vi "Test1_3.vi"(7 "Report Enable":bool, 8 "error in":errorcluster, 9 "Cycles Burst":i32=10000, 10 "DT_50_L0":i32[][](array[numeric]), 11 "Instrument VISA in":T1={"AWG VISA"="81160A", "Oscilloscope  VISA "="DSO80204B", "Integration Board IP"="172.16.7.43", "connection ID"=refnum, "report out"=refnum}) -> (0 "error out":errorcluster, 2 "L1_Calibration":dbl[][](array[numeric]), 3 "Instrument VISA out":T1={"AWG VISA"="81160A", "Oscilloscope  VISA "="DSO80204B", "Integration Board IP"="172.16.7.43", "connection ID"=refnum, "report out"=refnum})   [LabVIEW 2009]
doc: "This VI does a L1 calibration using different modes depending on the number of pixels active."
uses:
  <instrlib>/Agilent 81150/Agilent 81150.lvlib
  <vilib>/Analysis/NI_AALPro.lvlib
  <vilib>/Utility/NIReport.llb/NI_report.lvclass
  <vilib>/Utility/NIReport.llb/Append Text Table to Report (wrap).vi
  <vilib>/Utility/NIReport.llb/Append Report Text (str wrap).vi
panel:
  out "XY Graph":cluster{"Y":dbl[], "Y":dbl[]}[](graph)
  # "Mode"
  # "Row"
  # "Column"
  # "Number of pixels active"
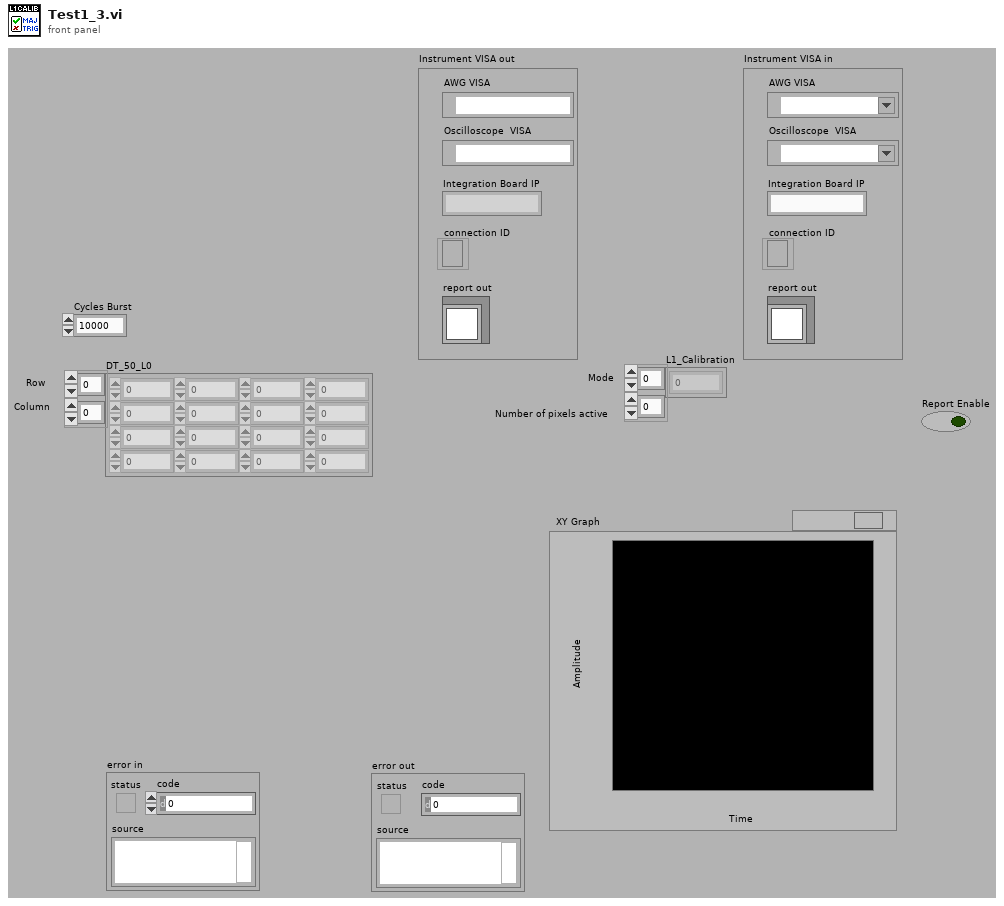
[diagram p1: front panel]
types:
  T1 = cluster{"AWG VISA":refnum<visa-resource-name>, "Oscilloscope  VISA ":refnum<visa-resource-name>, "Integration Board IP":string, "connection ID":refnum<k5>, "report out":refnum<class "NI_report.lvclass">}
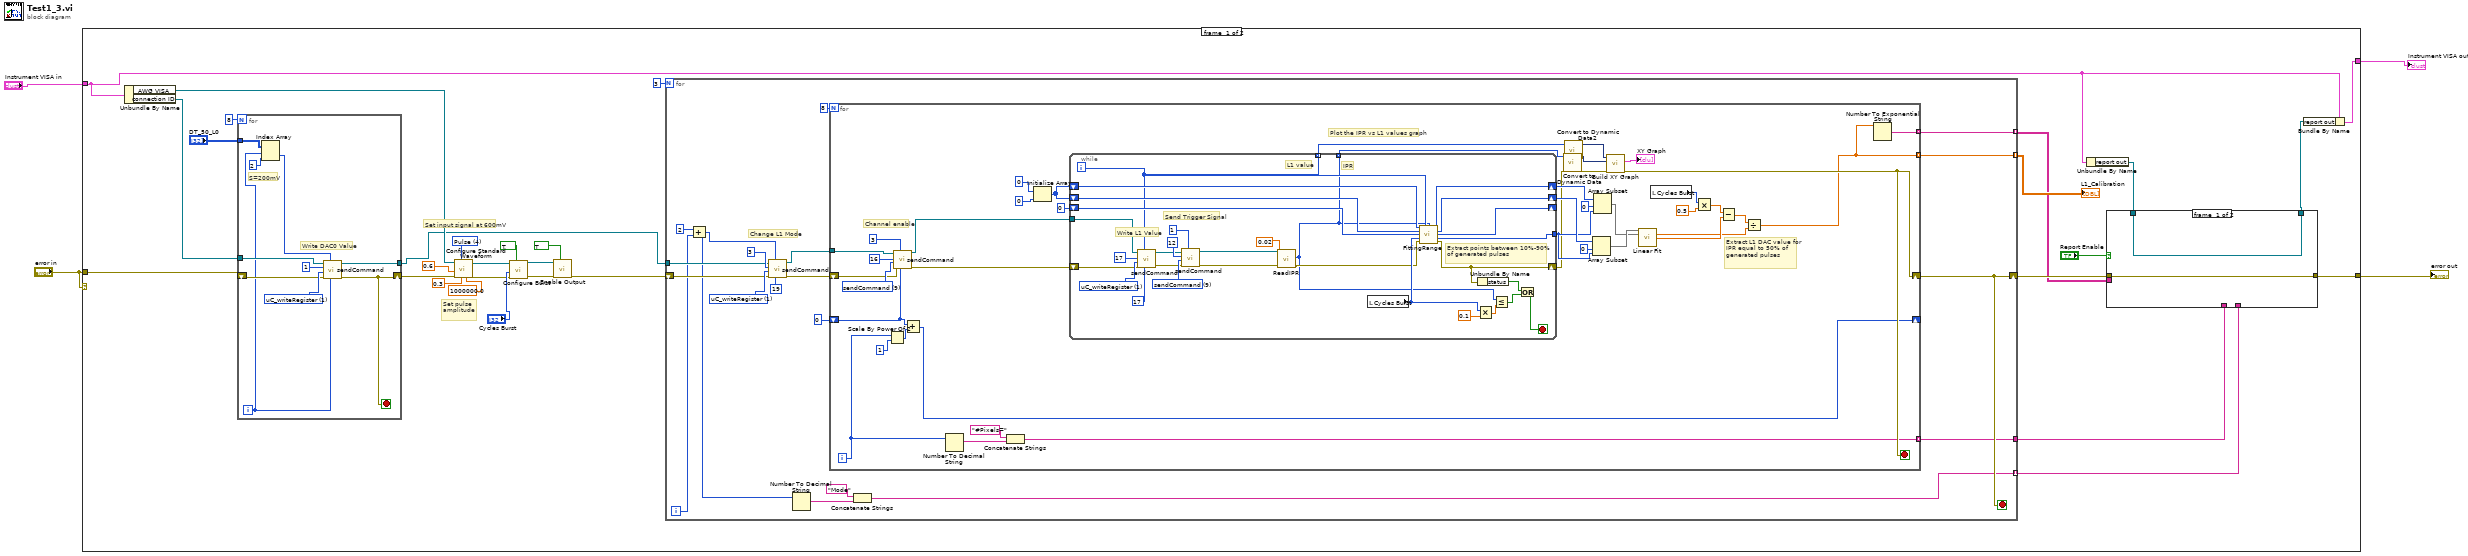
[diagram p0: block diagram]
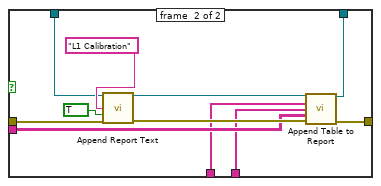
[diagram p2: hidden frame]
diagram:
  n1 = case shown="No Error" "error in" {
    tunnel: "error in" -> [w32 w150]
    tunnel: "Instrument VISA in" -> [w7 w149]
    tunnel: [w14 w150] -> w3
    tunnel: [w6 w149] -> w1
    frame #0 {
      w30 = u16 4 items=["Sine", "Square", "Ramp Up", "Ramp Down", "Pulse", "Noise", "DC"] ("Waveform (0: Sine)")
      # "Set input signal at 600mV"
      # "Set pulse amplitude"
      n2 = Unbundle By Name(w7) -> ("AWG VISA"=w27:refnum<visa-resource-name>, "connection ID"=w33:refnum<k5>)
      n3 = for {
        N: 8 -> [_]
        shift-right: [w139] -> w28
        shift-left: w32 -> [w145]
        tunnel: w33 -> [w143]
        tunnel: "DT_50_L0" -> [w146]
        tunnel: [w140] -> w17
        i -> [w141]
        stop <- w139 stop-if-true
        w148 = u16 1 items=["sendCommand"=9, "FPGA_writeRegister"=3, "FPGA_readRegister"=2, "uC_writeRegister"=1, "uC_readRegister"=0] ("Action")
        # "S=200mV"
        # "Write DAC0 Value"
        n4 = Index Array(array=w146, index (row)=w141, index (col)=2 ("disabled index (col)")) -> (element=w144:i32)
        n5 = call "sendCommand.vi"("Address"=w141, "Data"=w144, "error in"=w145, "Action"=w148, "id_in"=1 ("id"), "connection ID"=w143) -> ("error out"=w139:errorcluster, "connection ID out"=w140:refnum<k5>)  [unwired: 1 in, 3 out]
      }
      n6 = call <instrlib>:"Configure Standard Waveform.vi"("Frequency (1000.0 Hz)"=1000000.0, "DC Offset (0.0 Volts)"=0.3, "Waveform (0: Sine)"=w30, "error in (no error)"=w28, "Amplitude (1.0 Vpp)"=0.6, "VISA resource name"=w27) -> ("error out"=w21:errorcluster, "VISA resource name out"=w20:refnum<visa-resource-name>)  [unwired: 4 in]
      n7 = call <instrlib>:"Configure Burst.vi"("Enable Burst (F: Disable)"=TRUE, "error in (no error)"=w21, "Burst Count (2)"="Cycles Burst", "VISA resource name"=w20) -> ("error out"=w24:errorcluster, "VISA resource name out"=w23:refnum<visa-resource-name>)  [unwired: 6 in]
      n8 = call <instrlib>:"Enable Output.vi"("Enable Output (T: Enable)"=TRUE, "error in (no error)"=w24, "VISA resource name"=w23) -> ("error out"=w16:errorcluster)  [unwired: 7 in, 1 out]
      n9 = for {
        N: 3 -> [_]
        tunnel: [w60] -> w18 mode=indexing
        shift-right: [w59] -> w13
        shift-left: w16 -> [w58]
        tunnel: w17 -> [w57]
        tunnel: [w51] -> w12 mode=indexing
        tunnel: [w50] -> w11
        tunnel: [w49] -> w10 mode=indexing
        i -> [w55]
        stop <- w59 stop-if-true
        w67 = u16 1 items=["sendCommand"=9, "FPGA_writeRegister"=3, "FPGA_readRegister"=2, "uC_writeRegister"=1, "uC_readRegister"=0] ("Action")
        # "Change L1 Mode"
        n10 = Add(x=2, y=w55) -> (x+y=w52:i32)
        n11 = call "sendCommand.vi"("Address"=19, "Data"=w52, "error in"=w58, "Action"=w67, "id_in"=3 ("id"), "connection ID"=w57) -> ("error out"=w61:errorcluster, "connection ID out"=w62:refnum<k5>)  [unwired: 1 in, 3 out]
        n12 = Number To Decimal String(number=w52) -> (decimal integer string=w54:string)  [unwired: 1 in]
        n13 = for {
          N: 8 -> [_]
          tunnel: [w69] -> w60 mode=indexing
          shift-right: [w102] -> w59
          shift-left: w61 -> [w105]
          shift-right: [w98] -> _
          shift-left: 0 ("x") -> [w99]
          tunnel: w62 -> [w97]
          tunnel: [w70] -> w50 mode=indexing
          tunnel: [w68] -> w49 mode=indexing
          i -> [w71]
          stop <- w102 stop-if-true
          w108 = u16 9 items=["sendCommand"=9, "FPGA_writeRegister"=3, "FPGA_readRegister"=2, "uC_writeRegister"=1, "uC_readRegister"=0] ("Action")
          # "Extract L1 DAC value for IPR equal to 50% of generated pulses"
          # "Plot the IPR vs L1 values graph"
          # "Channel enable"
          n14 = Scale By Power Of 2(n=w71, x=1) -> (x*2^n=w100:i32)
          n15 = call "sendCommand.vi"("Address"=w99, "Data"=3, "error in"=w105, "Action"=w108, "id_in"=16 ("id"), "connection ID"=w97) -> ("error out"=w103:errorcluster, "connection ID out"=w101:refnum<k5>)  [unwired: 1 in, 3 out]
          n16 = Add(x=w99, y=w100) -> (x+y=w98:i32)
          n17 = Number To Decimal String(number=w71) -> (decimal integer string=w73:string)  [unwired: 1 in]
          n18 = Concatenate Strings("#Pixels=" ("string"), w73) -> (w70:string)
          n19 = Initialize Array(0 ("element"), 0 ("dimension size")) -> (w89:i32[])
          n20 = while {
            tunnel: [w109] -> w95 mode=indexing
            tunnel: [w126] -> w93 mode=indexing
            shift-right: [w133] -> w87
            shift-left: w89 -> [w131]
            shift-right: [w132] -> w86
            shift-left: w89 -> [w130]
            shift-right: [w122] -> w74
            shift-left: w103 -> [w136]
            shift-right: [w128] -> _
            shift-left: 0 ("Array Pointer out") -> [w129]
            tunnel: [w127] -> w83
            tunnel: w101 -> [w124]
            i -> [w126]
            stop <- w120 stop-if-true
            w116 = u16 9 items=["sendCommand"=9, "FPGA_writeRegister"=3, "FPGA_readRegister"=2, "uC_writeRegister"=1, "uC_readRegister"=0] ("Action")
            w138 = u16 1 items=["sendCommand"=9, "FPGA_writeRegister"=3, "FPGA_readRegister"=2, "uC_writeRegister"=1, "uC_readRegister"=0] ("Action")
            # "Send Trigger Signal"
            # "Extract points between 10%-90% of generated pulses"
            # "Write L1 Value"
            # "IPR"
            # "L1 value"
            n21 = call "sendCommand.vi"("Address"=17, "Data"=w126, "error in"=w136, "Action"=w138, "id_in"=17 ("id"), "connection ID"=w124) -> ("error out"=w115:errorcluster, "connection ID out"=w114:refnum<k5>)  [unwired: 1 in, 3 out]
            n22 = call "sendCommand.vi"("Data"=1, "error in"=w115, "Action"=w116, "id_in"=12 ("id"), "connection ID"=w114) -> ("error out"=w112:errorcluster, "connection ID out"=w110:refnum<k5>)  [unwired: 2 in, 3 out]
            n23 = call "ReadIPR.vi"("error in"=w112, 10:0.02 ("Delay Time (s)"), "connection ID"=w110) -> ("error out"=w111:errorcluster, "IPR value"=w109:i32)  [unwired: 6 in, 1 out]
            n24 = local read "Cycles Burst"() -> (w125:i32)
            n25 = call "FittingRange.vi"("Array in (X)"=w131, "L0 DAC"=w126, "IPR"=w109, "Array in (Y)"=w130, "Array Pointer in"=w129, "Cycles Burst"=w125, "error in"=w111) -> ("Array out (X)"=w133:i32[], "Array out (Y)"=w132:i32[], "Array Pointer out"=w128:i32, "N_Array Elements"=w127:i32, "error out"=w122:errorcluster)  [unwired: 4 in]
            n26 = Multiply(x=w125, y=0.1) -> (x*y=w134:dbl)
            n27 = Unbundle By Name(w122) -> ("status"=w121:bool)
            n28 = Less Or Equal?(x=w109, y=w134) -> (x <= y?=w123:bool)
            n29 = Or(x=w121, y=w123) -> (x .or. y?=w120:bool)
          }
          n30 = call "Convert to Dynamic Data"("Array"=w95) -> ("Dynamic Data Type"=w94:dynamicdata)  [unwired: 3 in]
          n31 = call "Convert to Dynamic Data2"("Array"=w93) -> ("Dynamic Data Type"=w92:dynamicdata)  [unwired: 3 in]
          n32 = Array Subset(array=w86, index=0, length=w83) -> (w82:i32[])
          n33 = Array Subset(array=w87, index=0, length=w83) -> (w81:i32[])
          n34 = call "Build XY Graph"("error in (no error)"=w74, "Y Input"=w94, "X Input"=w92) -> ("error out"=w102:errorcluster, "XY Graph"=→"XY Graph":cluster{"Y":dbl[], "Y":dbl[]}[])  [unwired: 7 in]
          n35 = call <vilib>:"Linear Fit.vi"("Y"=w82, "X"=w81) -> ("slope"=w75:dbl, "intercept"=w77:dbl)  [unwired: 9 in, 3 out]
          n36 = local read "Cycles Burst"() -> (w80:i32)
          n37 = Multiply(x=w80, y=0.5) -> (x*y=w78:dbl)
          n38 = Subtract(x=w78, y=w77) -> (x-y=w76:dbl)
          n39 = Divide(x=w76, y=w75) -> (x/y=w69:dbl)
          n40 = Number To Exponential String(number=w69) -> (E-format string=w68:string)  [unwired: 3 in]
        }
        n41 = Concatenate Strings("Mode" ("string"), w54) -> (w51:string)
      }
      "L1_Calibration" <- w18
      n42 = Unbundle By Name(w7) -> ("report out"=w9:refnum<class "NI_report.lvclass">)
      n43 = case shown="True" "Report Enable" {
        tunnel: [w36 w48] -> w14
        tunnel: w13 -> [w36 w47]
        tunnel: w9 -> [w37 w42]
        tunnel: w10 -> [_ w41]
        tunnel: w11 -> [_ w40]
        tunnel: w12 -> [_ w39]
        tunnel: [w37 w38] -> w8
        frame #0 {
        }
        frame #1 {
          n44 = call-poly <vilib>:"Append Report Text.vi"("report in"=w42, "text"="L1 Calibration", "append on new line? (F)"=TRUE, "error in (no error)"=w47) -> ("report out"=w43:refnum<class "NI_report.lvclass">, "error out"=w46:errorcluster)  [unwired: 8 in, 2 out]
          n45 = call-poly <vilib>:"Append Table to Report.vi"("report in"=w43, "column headers"=w40, "row headers"=w39, "text data"=w41, "error in (no error)"=w46) -> ("report out"=w38:refnum<class "NI_report.lvclass">, "error out"=w48:errorcluster)  [unwired: 7 in, 2 out]
        }
      }
      n46 = Bundle By Name(cluster=w7, "report out"=w8) -> (w6:T1)
    }
    frame #1 {
    }
  }
  "error out" <- w3
  "Instrument VISA out" <- w1
